vi "ReadAllPersonnel.vi"(8 "error in (no error)":errorcluster, 11 "PUID":string) -> (0 "error out":errorcluster, 1 "JSON":string, 2 "PersonnelJSON":string[](array[string]), 3 "Personnel":refnum<class "Personnel.lvclass">[](array[class]))   [LabVIEW 2015, in "PersonnelRestApi.lvlib"]
uses:
  PersonnelRestApi.lvlib
  LVClasses/Personnel/Personnel.lvclass
  TypeDef/GetPersonnelCommands.ctl
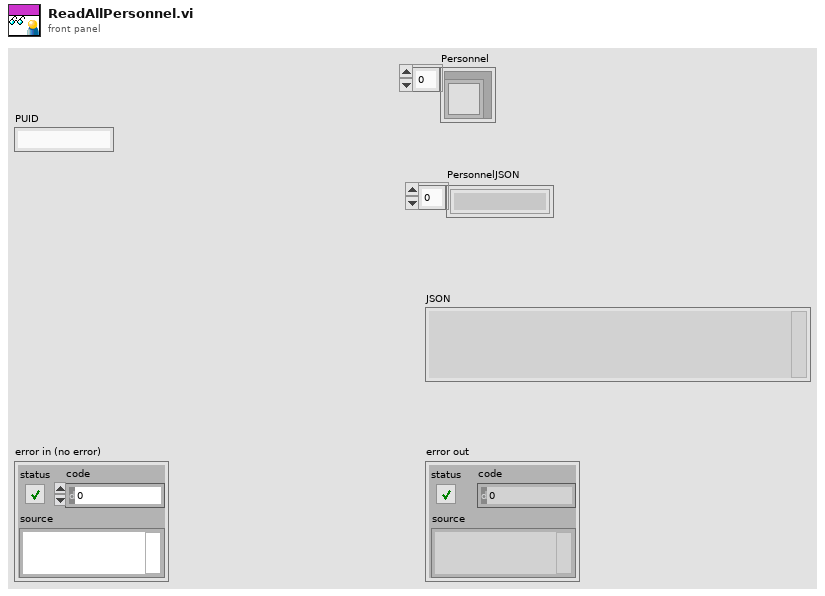
[diagram p1: front panel]
types:
  T1 = typedef "PersonnelRestApi.lvlib/GetPersonnelCommands.ctl" = enum16{"ReadPersonnel", "ReadName", "ReadRole", "ReadRequests", "ReadPUIDs", "ReadAllPersonnel"}
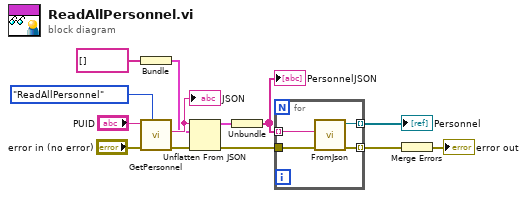
[diagram p0: block diagram]
diagram:
  n1 = Bundle("Personnel"=string[] []) -> (w6:cluster{"Personnel":string[]})  [unwired: 1 in]
  n2 = call "GetPersonnel.vi"("Room Commands"=GetPersonnelCommands."ReadAllPersonnel", "error in (no error)"="error in (no error)", "PUID"="PUID") -> ("error out"=w10:errorcluster, "JSON"=w9:string)  [unwired: 7 in]
  "JSON" <- w9
  n3 = Unflatten From JSON(JSON string=w9, type and defaults=w6, error in (no error)=w10) -> (value=w8:cluster{"Personnel":string[]}, error out=w2:errorcluster)  [unwired: 4 in]
  n4 = Unbundle(w8) -> ("Personnel"=w5:string[])
  "PersonnelJSON" <- w5
  n5 = for {
    tunnel: w5 -> [w17] mode=indexing
    tunnel: [w16] -> w3 mode=indexing
    tunnel: w2 -> [w15]
    tunnel: [w14] -> w1 mode=indexing
    n6 = call "FromJson.vi"("error in (no error)"=w15, "PersonnelJson"=w17) -> ("error out"=w16:errorcluster, "Personnel out"=w14:refnum<class "Personnel.lvclass">)  [unwired: 8 in]
  }
  "Personnel" <- w1
  n7 = Merge Errors(w3) -> (→"error out":errorcluster)
